vi "Main_Module.vi"(8 "Error In":errorcluster) -> (0 "Error Out":errorcluster)   [LabVIEW 2020]
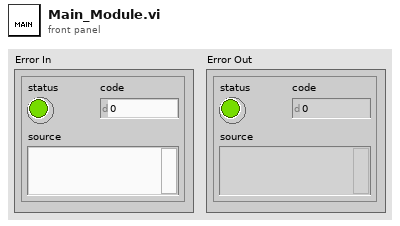
[diagram p1: front panel]
types:
  T1 = typedef "Queue.ctl" = cluster{"Mode":T2, "Data":variant}
  T2 = typedef "Queue_Mode.ctl" = enum16{"Start", "Stop"}
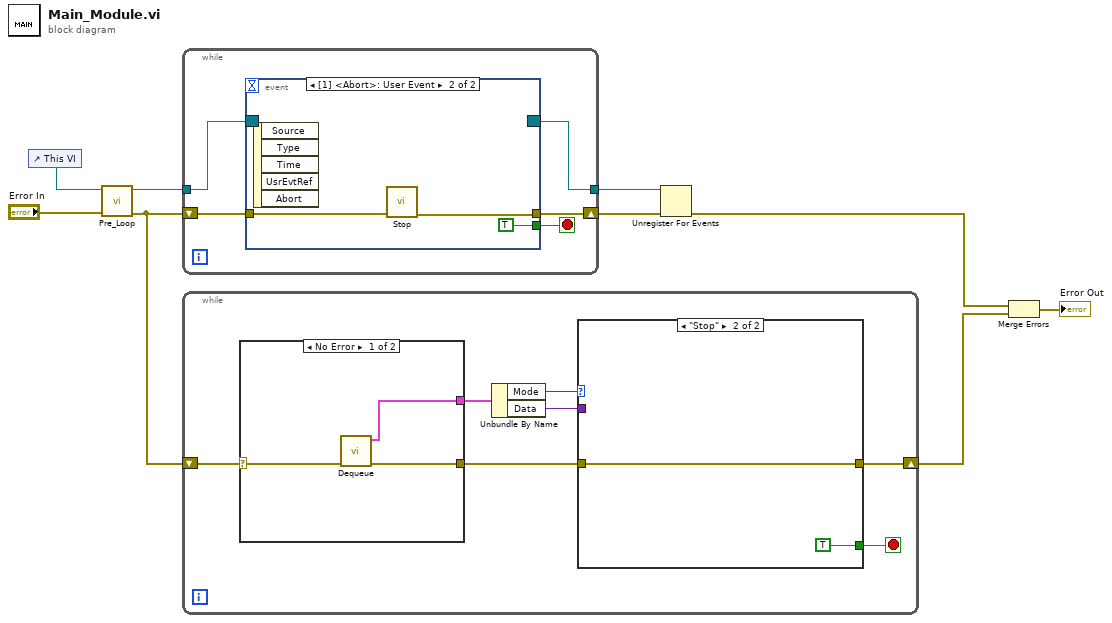
[diagram p0: block diagram]
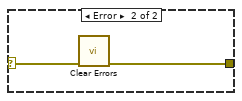
[diagram p3: hidden frame]
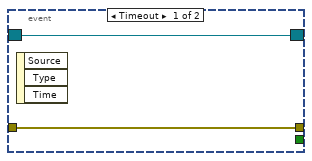
[diagram p4: hidden frame]
diagram:
  n1 = control-ref of="This VI"() -> (w8:refnum<vi>)
  n2 = call "Pre_Loop.vi"("Error In"="Error In", "This VI"=w8) -> ("Error Out"=w3:errorcluster, "Event Registration Refnum"=w7:refnum<event-registration>)  [unwired: 8 in]
  n3 = while {
    shift-right: [w11] -> w6
    shift-left: w3 -> [w14]
    tunnel: w7 -> [w13]
    tunnel: [w12] -> w5
    stop <- w10 stop-if-true
    n4 = event shown="[1] <Abort>: User Event" {
      selector: w13 -> [w16 _]
      dyn-events: [w16 _] -> w12
      timeout: _ -> [_ _]
      tunnel: w14 -> [w15 w19]
      tunnel: [w15 w18] -> w11
      tunnel: [_ TRUE] -> w10
      event Timeout {
        n5 = event-data() -> ()  [unwired: 1 in, 3 out]
      }
      event User Event {
        n6 = event-data() -> ()  [unwired: 1 in, 5 out]
        n7 = call "Stop.vi"("error in"=w19) -> ("error out"=w18:errorcluster)  [unwired: 10 in]
      }
    }
  }
  n8 = while {
    shift-right: [w20] -> w2
    shift-left: w3 -> [w26]
    stop <- w21 stop-if-true
    n9 = case shown="No Error" w26 {
      selector: w26 -> [w31 w33]
      tunnel: [w30 w32] -> w25
      tunnel: [w29 _] -> w24
      frame No Error {
        n10 = call "Dequeue.vi"("error in"=w31) -> ("error out"=w30:errorcluster, "element"=w29:T1)  [unwired: 9 in]
      }
      frame Error {
        n11 = call <vilib>:"Clear Errors.vi"("error in (no error)"=w33) -> ("error out"=w32:errorcluster)  [unwired: 5 in, 1 out]
      }
    }
    n12 = Unbundle By Name(w24) -> ("Mode"=w23:T2, "Data"=w22:variant)
    n13 = case shown="\"Stop\"" w23 {
      tunnel: w25 -> [_ w27]
      tunnel: w22 -> [_ _]
      tunnel: [_ TRUE] -> w21
      tunnel: [_ w27] -> w20
      frame "Start", Default {
      }
      frame "Stop" {
      }
    }
  }
  n14 = Unregister For Events(event registration refnum=w5, error in=w6) -> (error out=w1:errorcluster)
  n15 = Merge Errors(w1, w2) -> (→"Error Out":errorcluster)
